vi "Read Subpanel Ref.vi"(11 "Philips Subpanel in":refnum<class "Flex UI Subpanel.lvclass">) -> (2 "Subpanel Ref":refnum<vi>, 3 "Philips Subpanel out":refnum<class "Flex UI Subpanel.lvclass">)   [LabVIEW 2014, in "Flex UI Subpanel.lvclass"]
uses:
  Flex UI Subpanel.lvclass
  Flex UI Subpanel.lvclass/Flex UI Subpanel.ctl
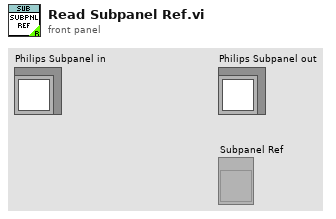
[diagram p1: front panel]
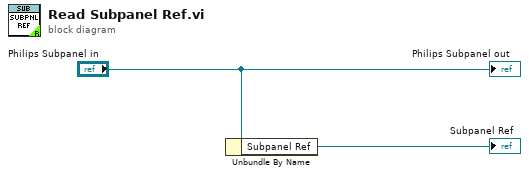
[diagram p0: block diagram]
diagram:
  n1 = Unbundle By Name("Philips Subpanel in") -> ("Subpanel Ref"=→"Subpanel Ref":refnum<vi>)
  "Philips Subpanel out" <- "Philips Subpanel in"
